vi "ExSubCreateFileStrip.vi"(2 "error in (no error)":errorcluster, 3 "File and Display Name":string, 4 "Pulser Handle":u32, 5 "Camera Handle":u32) -> (0 "error out":errorcluster, 1 "Handles Out":T1)   [LabVIEW 2010]
panel:
  # "ExSubCreateFileStrip:\nThis Sub-VI creates a file and opens it"
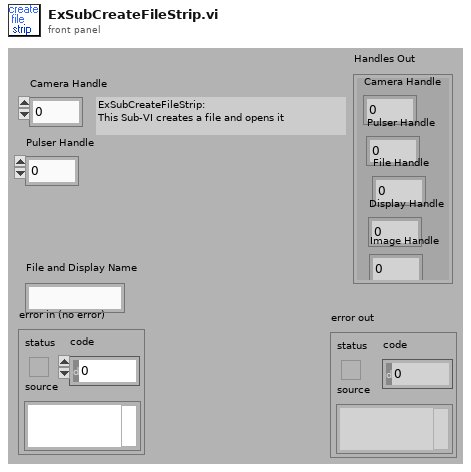
[diagram p1: front panel]
types:
  T1 = cluster{"Camera Handle":u32, "Pulser Handle":u32, "File Handle":u32, "Display Handle":u32, "Image Handle":u32}
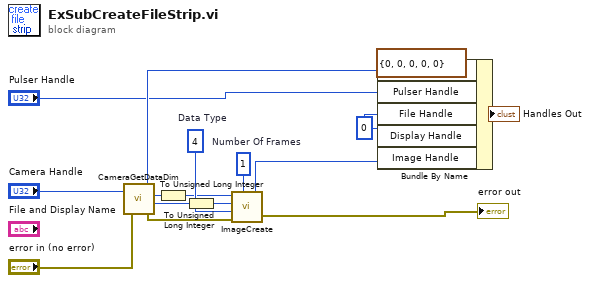
[diagram p0: block diagram]
diagram:
  w2 = u32 0 ("Display Handle")
  w9 = u32 4  # Data Type
  w10 = u32 1  # Number Of Frames
  n1 = call <userlib>:"CameraGetDataDim.vi"("Camera Handle"="Camera Handle", "error in"="error in (no error)") -> ("Camera Handle"=w8:u32, "Xdim"=w14:u32, "Ydim"=w15:u32, "error out"=w16:errorcluster)
  n2 = To Unsigned Long Integer(number=w14) -> (unsigned 32bit integer=w4:u32)
  n3 = To Unsigned Long Integer(number=w15) -> (unsigned 32bit integer=w3:u32)
  n4 = call <userlib>:"ImageCreate.vi"("X dimension"=w4, "Y dimension"=w3, "Data Type"=w9, "error in"=w16, "Number Of Frames"=w10) -> ("Image Handle"=w6:u32, "error out"=→"error out":errorcluster)
  n5 = Bundle By Name(cluster=T1 {"Camera Handle"=0, "Pulser Handle"=0, "File Handle"=0, "Display Handle"=0, "Image Handle"=0} ("Handles Out"), "Camera Handle"=w8, "Pulser Handle"="Pulser Handle", "File Handle"=w2, "Display Handle"=w2, "Image Handle"=w6) -> (→"Handles Out":T1)
